vi "ModeMgr.Populate All Options.vi"(9 "Options":string[](array[string])=["Can Access Station Module", "Can Auto Repeat Sequence", "Can Clear Errors", "Can Clear Warnings", "Can Edit EQ List", "Can Edit Options", "Can Generate Reports", "Can Open Data Folders", "Can Select Sequence", "Can View Config", "Disable Results", "Disable Start with SN Entry", "Display Result Data Details", "Not Reset SN between Tests", "Not Validate Operator", "Not Validate SN", "Display Result Data Details", "Not Reset SN between Tests", "Not Validate Operator", "Not Validate SN", "Disable Results", "Can Access Station Module", "Can Edit EQ List", "Can Clear Warnings", "Can Clear Errors", "Can View Config", "Can Edit Options", "Can Select Sequence", "Can Generate Reports", "Disable Start with SN Entry", "Can Auto Repeat Sequence"], 11 "Modes":T1[](array[typedef])=[{"Name"="", "Color"=0, "Options"=[{"Option"="Display Result Data Details", "Level"=0}, {"Option"="Not Reset SN between Tests", "Level"=0}, {"Option"="Not Validate Operator", "Level"=0}, {"Option"="Not Validate SN", "Level"=0}, {"Option"="Disable Results", "Level"=0}, {"Option"="Can Access Station Module", "Level"=0}, {"Option"="Can Edit EQ List", "Level"=0}, {"Option"="Can Clear Warnings", "Level"=0}, {"Option"="Can Clear Errors", "Level"=0}, {"Option"="Can View Config", "Level"=0}, {"Option"="Can Edit Options", "Level"=0}, {"Option"="Can Select Sequence", "Level"=0}, {"Option"="Can Generate Reports", "Level"=0}, {"Option"="Disable Start with SN Entry", "Level"=0}], "Password"=""}, {"Name"="", "Color"=0, "Options"=[{"Option"="Display Result Data Details", "Level"=0}, {"Option"="Not Reset SN between Tests", "Level"=0}, {"Option"="Not Validate Operator", "Level"=0}, {"Option"="Not Validate SN", "Level"=0}, {"Option"="Disable Results", "Level"=0}, {"Option"="Can Access Station Module", "Level"=0}, {"Option"="Can Edit EQ List", "Level"=0}, {"Option"="Can Clear Warnings", "Level"=0}, {"Option"="Can Clear Errors", "Level"=0}, {"Option"="Can View Config", "Level"=0}, {"Option"="Can Edit Options", "Level"=0}, {"Option"="Can Select Sequence", "Level"=0}, {"Option"="Can Generate Reports", "Level"=0}, {"Option"="Disable Start with SN Entry", "Level"=0}], "Password"=""}, {"Name"="", "Color"=0, "Options"=[{"Option"="Display Result Data Details", "Level"=0}, {"Option"="Not Reset SN between Tests", "Level"=0}, {"Option"="Not Validate Operator", "Level"=0}, {"Option"="Not Validate SN", "Level"=0}, {"Option"="Disable Results", "Level"=0}, {"Option"="Can Access Station Module", "Level"=0}, {"Option"="Can Edit EQ List", "Level"=0}, {"Option"="Can Clear Warnings", "Level"=0}, {"Option"="Can Clear Errors", "Level"=0}, {"Option"="Can View Config", "Level"=0}, {"Option"="Can Edit Options", "Level"=0}, {"Option"="Can Select Sequence", "Level"=0}, {"Option"="Can Generate Reports", "Level"=0}, {"Option"="Disable Start with SN Entry", "Level"=0}], "Password"=""}, {"Name"="", "Color"=0, "Options"=[{"Option"="Display Result Data Details", "Level"=0}, {"Option"="Not Reset SN between Tests", "Level"=0}, {"Option"="Not Validate Operator", "Level"=0}, {"Option"="Not Validate SN", "Level"=0}, {"Option"="Disable Results", "Level"=0}, {"Option"="Can Access Station Module", "Level"=0}, {"Option"="Can Edit EQ List", "Level"=0}, {"Option"="Can Clear Warnings", "Level"=0}, {"Option"="Can Clear Errors", "Level"=0}, {"Option"="Can View Config", "Level"=0}, {"Option"="Can Edit Options", "Level"=0}, {"Option"="Can Select Sequence", "Level"=0}, {"Option"="Can Generate Reports", "Level"=0}, {"Option"="Disable Start with SN Entry", "Level"=0}], "Password"=""}] {"Color" items=["Red", "Yellow", "Orange", "Green", "SkyBlue", "Blue", "Purple", "Pink", "Grey"]}) -> (3 "Modes Out":T1[](array[typedef])=[{"Name"="", "Color"=0, "Options"=[{"Option"="Display Result Data Details", "Level"=0}, {"Option"="Not Reset SN between Tests", "Level"=0}, {"Option"="Not Validate Operator", "Level"=0}, {"Option"="Not Validate SN", "Level"=0}, {"Option"="Disable Results", "Level"=0}, {"Option"="Can Access Station Module", "Level"=0}, {"Option"="Can Edit EQ List", "Level"=0}, {"Option"="Can Clear Warnings", "Level"=0}, {"Option"="Can Clear Errors", "Level"=0}, {"Option"="Can View Config", "Level"=0}, {"Option"="Can Edit Options", "Level"=0}, {"Option"="Can Select Sequence", "Level"=0}, {"Option"="Can Generate Reports", "Level"=0}, {"Option"="Disable Start with SN Entry", "Level"=0}], "Password"=""}, {"Name"="", "Color"=0, "Options"=[{"Option"="Display Result Data Details", "Level"=0}, {"Option"="Not Reset SN between Tests", "Level"=0}, {"Option"="Not Validate Operator", "Level"=0}, {"Option"="Not Validate SN", "Level"=0}, {"Option"="Disable Results", "Level"=0}, {"Option"="Can Access Station Module", "Level"=0}, {"Option"="Can Edit EQ List", "Level"=0}, {"Option"="Can Clear Warnings", "Level"=0}, {"Option"="Can Clear Errors", "Level"=0}, {"Option"="Can View Config", "Level"=0}, {"Option"="Can Edit Options", "Level"=0}, {"Option"="Can Select Sequence", "Level"=0}, {"Option"="Can Generate Reports", "Level"=0}, {"Option"="Disable Start with SN Entry", "Level"=0}], "Password"=""}, {"Name"="", "Color"=0, "Options"=[{"Option"="Display Result Data Details", "Level"=0}, {"Option"="Not Reset SN between Tests", "Level"=0}, {"Option"="Not Validate Operator", "Level"=0}, {"Option"="Not Validate SN", "Level"=0}, {"Option"="Disable Results", "Level"=0}, {"Option"="Can Access Station Module", "Level"=0}, {"Option"="Can Edit EQ List", "Level"=0}, {"Option"="Can Clear Warnings", "Level"=0}, {"Option"="Can Clear Errors", "Level"=0}, {"Option"="Can View Config", "Level"=0}, {"Option"="Can Edit Options", "Level"=0}, {"Option"="Can Select Sequence", "Level"=0}, {"Option"="Can Generate Reports", "Level"=0}, {"Option"="Disable Start with SN Entry", "Level"=0}], "Password"=""}, {"Name"="", "Color"=0, "Options"=[{"Option"="Display Result Data Details", "Level"=0}, {"Option"="Not Reset SN between Tests", "Level"=0}, {"Option"="Not Validate Operator", "Level"=0}, {"Option"="Not Validate SN", "Level"=0}, {"Option"="Disable Results", "Level"=0}, {"Option"="Can Access Station Module", "Level"=0}, {"Option"="Can Edit EQ List", "Level"=0}, {"Option"="Can Clear Warnings", "Level"=0}, {"Option"="Can Clear Errors", "Level"=0}, {"Option"="Can View Config", "Level"=0}, {"Option"="Can Edit Options", "Level"=0}, {"Option"="Can Select Sequence", "Level"=0}, {"Option"="Can Generate Reports", "Level"=0}, {"Option"="Disable Start with SN Entry", "Level"=0}], "Password"=""}] {"Color" items=["Red", "Yellow", "Orange", "Green", "SkyBlue", "Blue", "Purple", "Pink", "Grey"]})   [LabVIEW 2018]
uses:
  ModeMgr.Mode Settings_Config View.ctl
  ModeMgr.Mode Settings.ctl
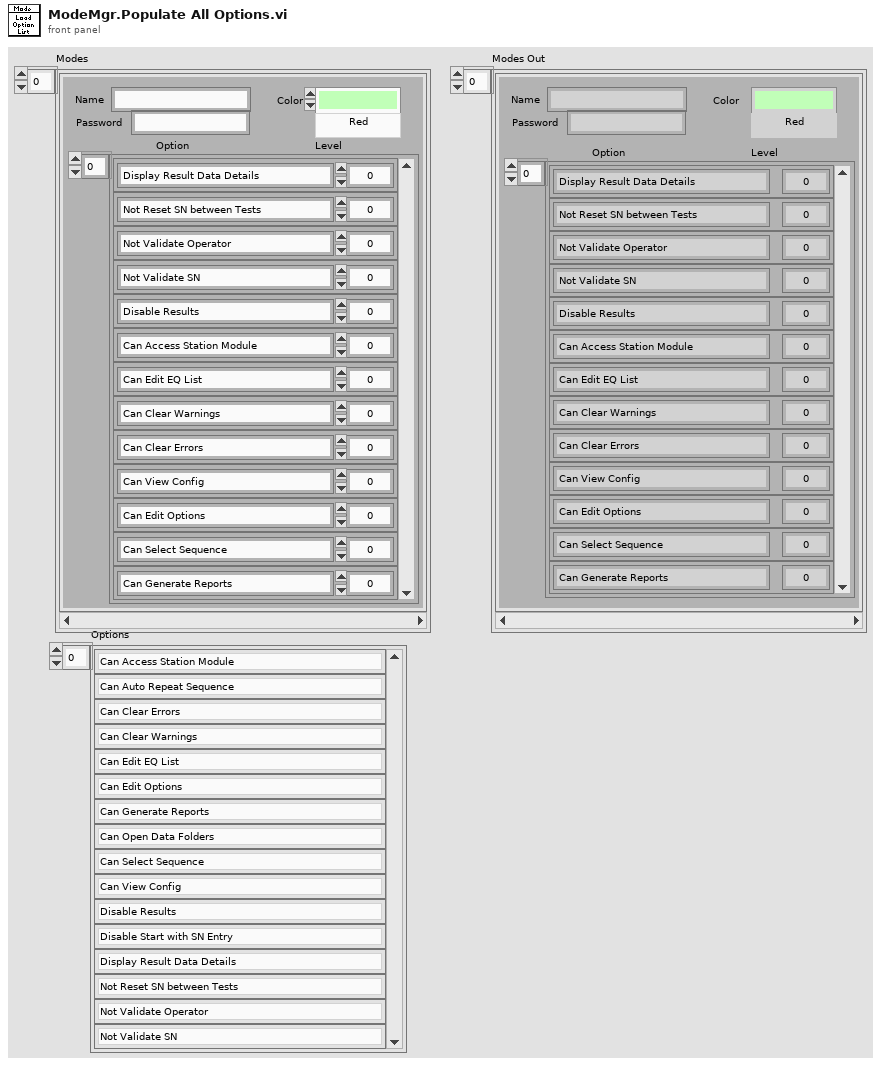
[diagram p1: front panel]
types:
  T1 = typedef "ModeMgr.Mode Settings_Config View.ctl" = cluster{"Name":string, "Color":u16, "Options":T2[], "Password":string}
  T2 = typedef "ModeMgr.Mode Settings.ctl" = cluster{"Option":string, "Level":i32}
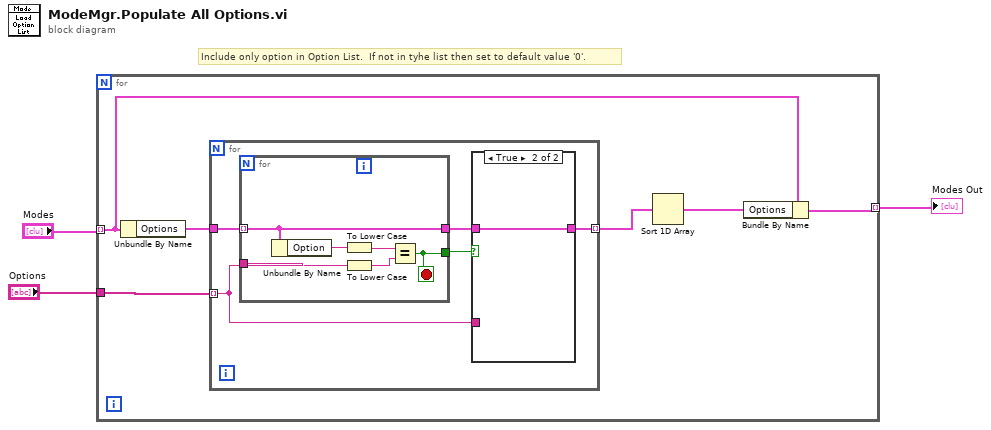
[diagram p0: block diagram]
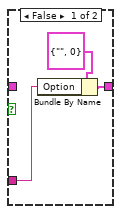
[diagram p2: hidden frame]
diagram:
  # "Include only option in Option List.  If not in tyhe list then set to default value '0'."
  n1 = for {
    tunnel: "Modes" -> [w8] mode=indexing
    tunnel: "Options" -> [w9]
    tunnel: [w6] -> w1 mode=indexing
    n2 = Unbundle By Name(w8) -> ("Options"=w5:T2[])
    n3 = for {
      tunnel: w9 -> [w11] mode=indexing
      tunnel: w5 -> [w14]
      tunnel: [w10] -> w4 mode=indexing
      n4 = for {
        tunnel: w14 -> [w23] mode=indexing
        tunnel: w11 -> [w19]
        tunnel: [w24] -> w13
        tunnel: [w23] -> w12
        stop <- w24 stop-if-true
        n5 = Unbundle By Name(w23) -> ("Option"=w22:string)
        n6 = To Lower Case(string=w22) -> (all lower case string=w21:string)
        n7 = To Lower Case(string=w19) -> (all lower case string=w20:string)
        n8 = Equal?(x=w21, y=w20) -> (x = y?=w24:bool)
      }
      n9 = case shown="True" w13 {
        tunnel: w12 -> [_ w18]
        tunnel: w11 -> [w15 _]
        tunnel: [w16 w18] -> w10
        frame False {
          n10 = Bundle By Name(cluster=T2 {"Option"="", "Level"=0} ("Setting"), "Option"=w15) -> (w16:T2)
        }
        frame True {
        }
      }
    }
    n11 = Sort 1D Array(array=w4) -> (sorted array=w7:T2[])
    n12 = Bundle By Name(cluster=w8, "Options"=w7) -> (w6:T1)
  }
  "Modes Out" <- w1
